vi "clear_job.vi"(8 "error in (no error)":errorcluster, 10 "job queue":refnum<queue>, 11 "job paths":path[](array[path])) -> (0 "error out":errorcluster, 3 "job paths out":path[](array[path]))   [LabVIEW 2024, in "Download_Manager.lvlib"]
uses:
  Download_Manager.lvlib
  typedefs/job--cluster.ctl
  typedefs/job_type--enum.ctl
panel:
  out "deleted portion":path
  out "# elements in queue":i32
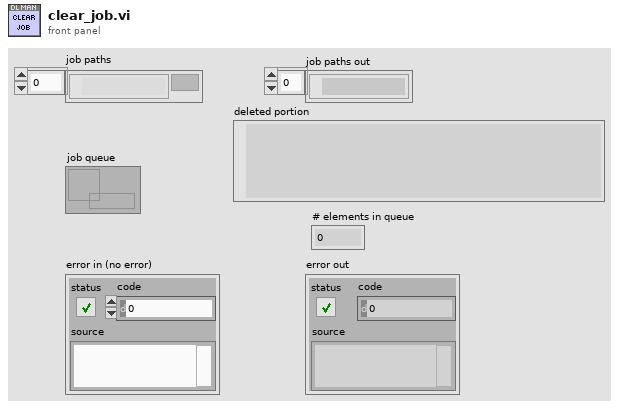
[diagram p1: front panel]
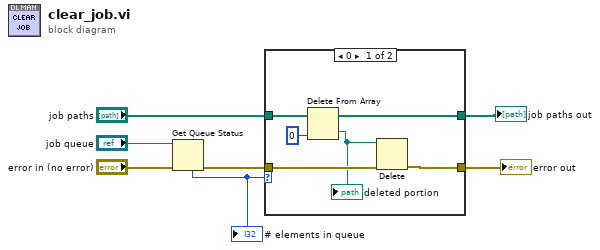
[diagram p0: block diagram]
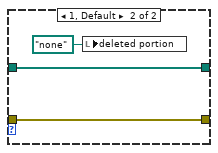
[diagram p2: hidden frame]
diagram:
  n1 = Get Queue Status(queue="job queue", error in (no error)="error in (no error)") -> (error out=w2:errorcluster, # elements in queue=w5:i32)  [unwired: 1 in, 6 out]
  "# elements in queue" <- w5
  n2 = case shown="0" w5 {
    tunnel: "job paths" -> [w13 w16]
    tunnel: [w11 w16] -> w3
    tunnel: w2 -> [w10 w15]
    tunnel: [w8 w15] -> w1
    frame 0 {
      n3 = Delete From Array(array=w13, index=0) -> (deleted portion=w9:path, array with subset deleted=w11:path[])  [unwired: 1 in]
      "deleted portion" <- w9
      n4 = Delete(path (use dialog)=w9, error in=w10) -> (error out=w8:errorcluster)  [unwired: 3 in, 2 out]
    }
    frame 1, Default {
      n5 = local write "deleted portion"(path "none" ("deleted portion")) -> ()
    }
  }
  "error out" <- w1
  "job paths out" <- w3
